vi "ADAM_Server_Channels.vi"() -> ()   [LabVIEW 2013]
uses:
  ADAM Client/Sub VIs/ADAM Controls/Search_mode.ctl
  <vilib>/Analysis/baseanly.llb/Mean (DBL).vi
  Globals/Meas_global.vi
  <vilib>/Analysis/NI_AALBase.lvlib
panel:
  out "Waveform Graph":dbl[][](graph)
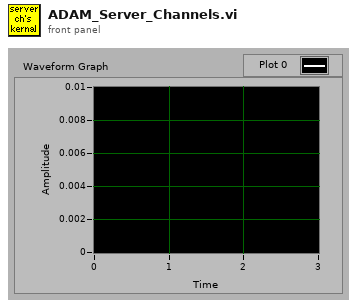
[diagram p1: front panel]
types:
  T1 = typedef "Analysis_info_cluster.ctl" = cluster{"Colour":u32, "Inst type":T2, "Inst name":string, "Symbol":string, "Code name":string, "Extra Info":string, "Inst Array":T3, "Extra Titles":string[], "Extra Values":string[], "U":dbl, "u^2":dbl, "u^3":dbl, "u^4":dbl, "Skew_u":dbl, "Kurt_u":dbl, "Sd Error in Mean":dbl, "% u'/U":dbl, "X":dbl, "Y":dbl, "Z":dbl, "Timescale integral to 25%":dbl, "Sd Error in Variance":dbl, "Calib File":path, "Calib Constants":dbl[], "Output Position":bool, "Full Stats":bool, "Av Sampling Rate":dbl, "Av No of Samples":dbl, "Total Meas Time (s)":dbl, "ADAM Ch Name":string}
  T2 = typedef "Inst_type.ctl" = enum16{"Propeller anemometer", "Raw voltage", "Pressure Transducer", "Pitot-static tube", "Preston tube", "Hot wire", "Cross wire 1", "Cross wire 2", "Generic Linear", "Generic Polynomial", "Generic BackPoly", "Fast FID", "Thermocouple", "Cold wire", "Pulsed Wire", "LDA Vel", "LDA Tran time", "LDA Arr time"}
  T3 = typedef "Instrument_Array.ctl" = enum16{"PWA", "LDA", "Analogue"}
  T4 = typedef "Search_mode.ctl" = enum16{"Between times", "All Times"}
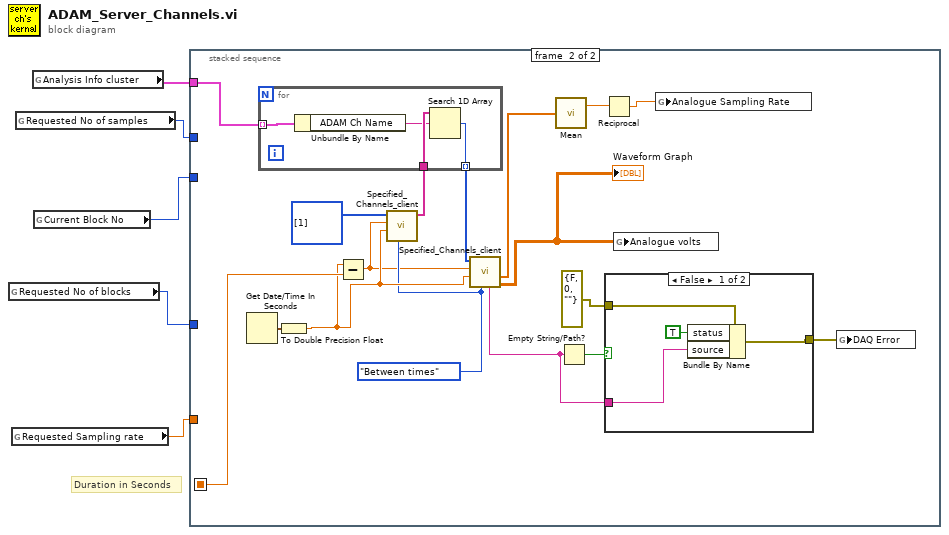
[diagram p0: block diagram]
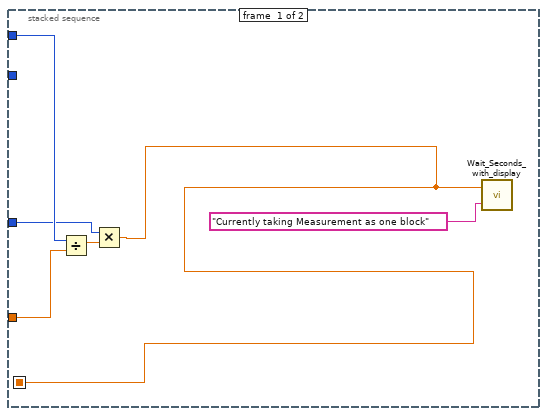
[diagram p2: hidden frame]
diagram:
  # "Duration in Seconds"
  n1 = global read "Meas_global.vi" "Requested No of blocks"() -> (w1:i32)
  n2 = global read "Meas_global.vi" "Requested Sampling rate"() -> (w4:dbl)
  n3 = global read "Meas_global.vi" "Requested No of samples"() -> (w5:i32)
  n4 = global read "Meas_global.vi" "Analysis Info cluster"() -> (w2:T1[])
  n5 = global read "Meas_global.vi" "Current Block No"() -> (w3:i32)
  n6 = stacked-sequence {
    seq-local: [w6 _] -> [_ w27]
    tunnel: w5 -> [w11 _]
    tunnel: w3 -> [_ _]
    tunnel: w2 -> [_ w19]
    tunnel: w4 -> [w10 _]
    tunnel: w1 -> [w8 _]
    frame #0 {
      n7 = Divide(x=w11, y=w10) -> (x/y=w9:dbl)
      n8 = Multiply(x=w8, y=w9) -> (x*y=w6:dbl)
      n9 = call "Wait_Seconds_with_display.vi"("Message"="Currently taking Measurement as one block", "Seconds to wait"=w6) -> ()  [unwired: 2 out]
    }
    frame #1 {
      w22 = Search_mode."Between times" ("Mode")
      n10 = Get Date/Time In Seconds() -> (seconds since 1Jan1904=w28:timestamp)
      n11 = To Double Precision Float(number=w28) -> (double precision float=w26:dbl)
      n12 = Subtract(x=w26, y=w27) -> (x-y=w21:dbl)
      n13 = call "Specified_Channels_client.vi"("Mode"=w22, "End time"=w26, "Start time"=w21, "ADAM Index array"=i32[] [1]) -> ("All Active Ch Names"=w24:string[])  [unwired: 1 in, 6 out]
      n14 = for {
        tunnel: w19 -> [w37] mode=indexing
        tunnel: w24 -> [w36]
        tunnel: [w34] -> w23 mode=indexing
        n15 = Unbundle By Name(w37) -> ("ADAM Ch Name"=w35:string)
        n16 = Search 1D Array(1D array=w36, element=w35) -> (index of element=w34:i32)  [unwired: 1 out]
      }
      n17 = call "Specified_Channels_client.vi"("Mode"=w22, "End time"=w26, "Start time"=w21, "ADAM Index array"=w23) -> ("Output array"=w20:dbl[][], "Averaging Period"=w18:dbl[], "Messages"=w12:string)  [unwired: 1 in, 4 out]
      "Waveform Graph" <- w20
      n18 = call-poly <vilib>:"Mean.vi"("X"=w18) -> ("mean"=w17:dbl)  [unwired: 1 out]
      n19 = Empty String/Path?(string/path=w12) -> (empty?=w15:bool)
      n20 = Reciprocal(x=w17) -> (1/x=w16:dbl)
      n21 = case shown="False" w15 {
        tunnel: errorcluster {"status"=FALSE, "code"=0, "source"=""} ("DAQ Error") -> [w32 w33]
        tunnel: [w31 w33] -> w13
        tunnel: w12 -> [w29 _]
        frame False {
          n22 = Bundle By Name(cluster=w32, "status"=TRUE, "source"=w29) -> (w31:errorcluster)
        }
        frame True {
        }
      }
      n23 = global write "Meas_global.vi" "Analogue volts"(w20) -> ()
      n24 = global write "Meas_global.vi" "Analogue Sampling Rate"(w16) -> ()
      n25 = global write "Meas_global.vi" "DAQ Error"(w13) -> ()
    }
  }
